vi "Parse Status Code from Headers String.vi"(11 "headers in":string) -> (2 "status code":u32)   [LabVIEW 2020, in "HTTP Client Abstract.lvlib" / "Abstract HTTP Client.lvclass"]
uses:
  Abstract HTTP Client.lvclass
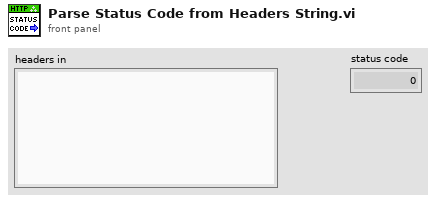
[diagram p1: front panel]
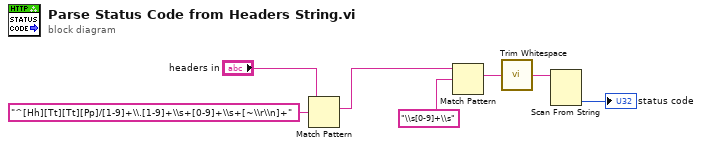
[diagram p0: block diagram]
diagram:
  n1 = Match Pattern(string="headers in", regular expression="^[Hh][Tt][Tt][Pp]/[1-9]+\\.[1-9]+\\s+[0-9]+\\s+[~\\r\\n]+") -> (match substring=w1:string)  [unwired: 1 in, 3 out]
  n2 = Match Pattern(string=w1, regular expression="\\s[0-9]+\\s") -> (match substring=w6:string)  [unwired: 1 in, 3 out]
  n3 = call <vilib>:"Trim Whitespace.vi"("string"=w6) -> ("trimmed string"=w5:string)  [unwired: 1 in]
  n4 = Scan From String(input string=w5) -> (output 1=→"status code":u32)  [unwired: 4 in, 3 out]
